vi "Parse Mail Header Info.vi"(0 "Message Content":string, 1 "error in (no error)":errorcluster) -> (2 "Date":string, 3 "Subject":string, 4 "Message Content out":string, 5 "To":string, 6 "From":string, 7 "error out":errorcluster)   [LabVIEW 2012]
doc: "This VI takes the full text of a message and parses through the header information to locate the Subject, From, To, and Date fields."
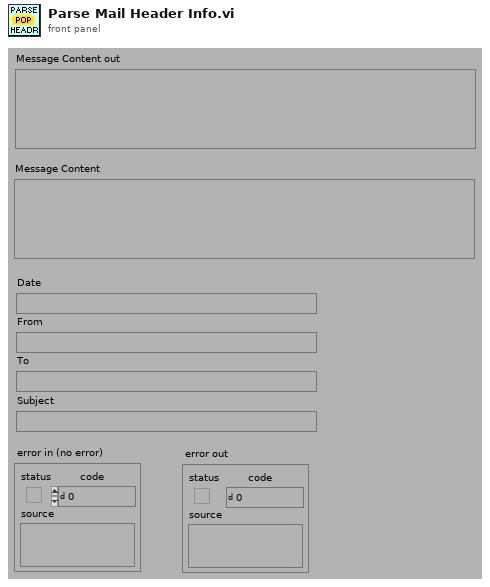
[diagram p1: front panel]
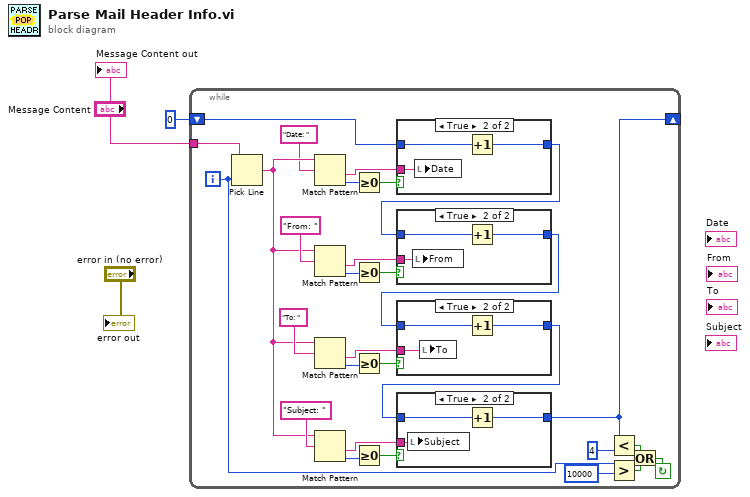
[diagram p0: block diagram]
diagram:
  n1 = while {
    shift-left: 0 -> [w23]
    shift-right: [w9] -> _
    tunnel: "Message Content" -> [w32]
    i -> [w7]
    stop <- w4 continue-if-true
    n2 = Pick Line(multi-line string=w32, line index=w7) -> (output string=w28:string)  [unwired: 1 in]
    n3 = Match Pattern(string=w28, regular expression="Date: ") -> (after substring=w24:string, offset past match=w27:i32)  [unwired: 1 in, 2 out]
    n4 = Match Pattern(string=w28, regular expression="From: ") -> (after substring=w18:string, offset past match=w19:i32)  [unwired: 1 in, 2 out]
    n5 = Match Pattern(string=w28, regular expression="To: ") -> (after substring=w16:string, offset past match=w17:i32)  [unwired: 1 in, 2 out]
    n6 = Match Pattern(string=w28, regular expression="Subject: ") -> (after substring=w14:string, offset past match=w15:i32)  [unwired: 1 in, 2 out]
    n7 = Greater Or Equal To 0?(x=w27) -> (x >= 0?=w26:bool)
    n8 = Greater Or Equal To 0?(x=w19) -> (x >= 0?=w22:bool)
    n9 = Greater Or Equal To 0?(x=w17) -> (x >= 0?=w21:bool)
    n10 = Greater Or Equal To 0?(x=w15) -> (x >= 0?=w20:bool)
    n11 = case shown="True" w26 {
      tunnel: w24 -> [_ w48]
      tunnel: w23 -> [w45 w47]
      tunnel: [w45 w46] -> w13
      frame False {
      }
      frame True {
        n12 = local write "Date"(w48) -> ()
        n13 = Increment(x=w47) -> (x+1=w46:i32)
      }
    }
    n14 = case shown="True" w22 {
      tunnel: w18 -> [_ w44]
      tunnel: w13 -> [w41 w43]
      tunnel: [w41 w42] -> w12
      frame False {
      }
      frame True {
        n15 = local write "From"(w44) -> ()
        n16 = Increment(x=w43) -> (x+1=w42:i32)
      }
    }
    n17 = case shown="True" w21 {
      tunnel: w16 -> [_ w40]
      tunnel: w12 -> [w37 w39]
      tunnel: [w37 w38] -> w11
      frame False {
      }
      frame True {
        n18 = local write "To"(w40) -> ()
        n19 = Increment(x=w39) -> (x+1=w38:i32)
      }
    }
    n20 = case shown="True" w20 {
      tunnel: w14 -> [_ w36]
      tunnel: w11 -> [w33 w35]
      tunnel: [w33 w34] -> w9
      frame False {
      }
      frame True {
        n21 = local write "Subject"(w36) -> ()
        n22 = Increment(x=w35) -> (x+1=w34:i32)
      }
    }
    n23 = Less?(x=w9, y=4) -> (x < y?=w6:bool)
    n24 = Greater?(x=w7, y=10000) -> (0:w5:bool)
    n25 = Or(x=w6, y=w5) -> (x .or. y?=w4:bool)
  }
  "Message Content out" <- "Message Content"
  "error out" <- "error in (no error)"
